vi "Handle Reply Msg.vi"(8 "error in (no error)":errorcluster, 9 "Panel Controller":refnum<class "Panel Controller Interface.lvclass">, 10 "EditPanel API in":refnum<class "EditPanel API.lvclass">, 11 "Console Error(Console2API) in":refnum<class "Console Reply Error Report.lvclass">) -> (0 "error out":errorcluster, 2 "EditPanel API out":refnum<class "EditPanel API.lvclass">)   [LabVIEW 2015, in "EditPanel API.lvlib" / "Console Reply Error Report.lvclass"]
uses:
  Console Reply Error Report.lvclass
  EditPanel_class/EditPanel API.lvclass
  Panel Control_Interface/Panel_interface/Panel Controller Interface.lvclass
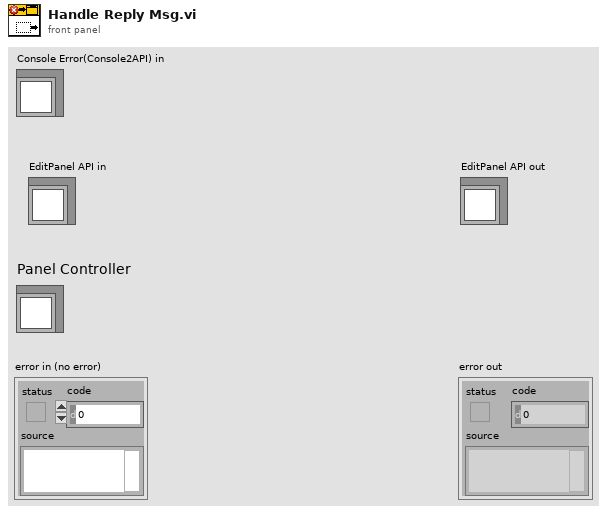
[diagram p1: front panel]
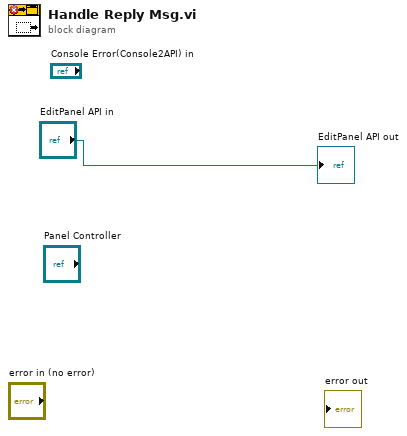
[diagram p0: block diagram]
diagram:
  "EditPanel API out" <- "EditPanel API in"
